vi "picoquant_datalog_loop.vi"(8 "error in (no error)":errorcluster, 11 "picoquant_generic in":refnum<class "picoquant_generic.lvclass">) -> (0 "error out":errorcluster, 3 "picoquant_generic out":refnum<class "picoquant_generic.lvclass">)   [LabVIEW 2015, in "picoquant_generic.lvclass"]
uses:
  picoquant_generic.lvclass
  picoquant_generic.lvclass/picoquant_generic.ctl
  loop_notifier_tdef.ctl
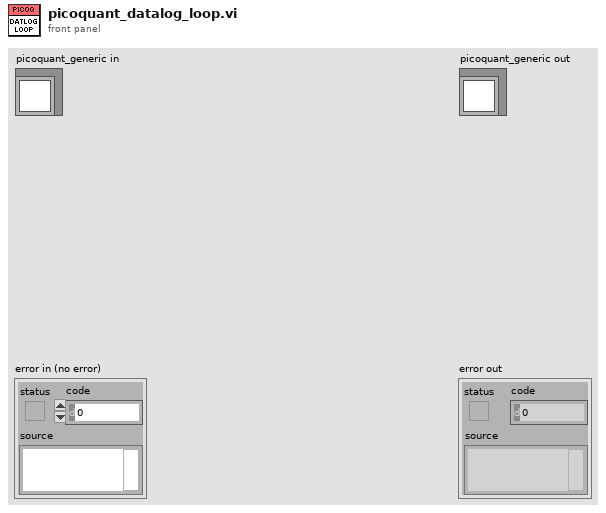
[diagram p1: front panel]
types:
  T1 = typedef "loop_notifier_tdef.ctl" = enum16{"exit"}
  T2 = typedef "picoquant_data_tdef.ctl" = cluster{"channels":u8[], "times":u64[], "sync":u64[]}
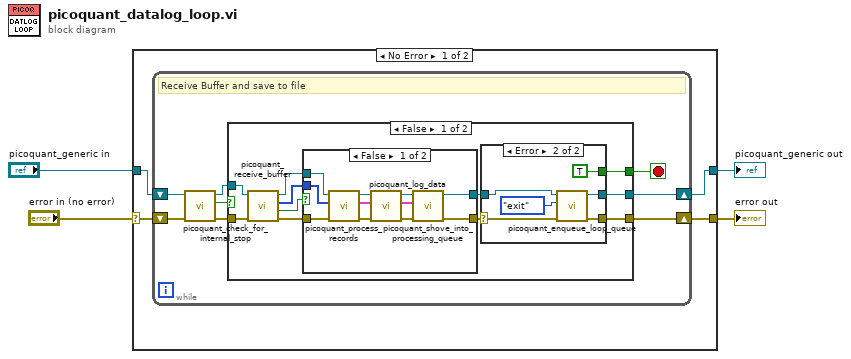
[diagram p0: block diagram]
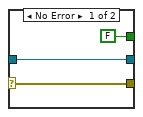
[diagram p2: hidden frame]
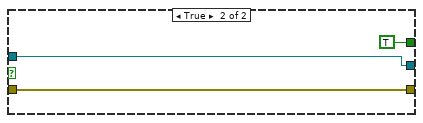
[diagram p4: hidden frame]
diagram:
  n1 = case shown="No Error" "error in (no error)" {
    selector: "error in (no error)" -> [w7 w54]
    tunnel: [w6 w54] -> w3
    tunnel: [w5 w53] -> w1
    tunnel: "picoquant_generic in" -> [w8 w53]
    frame No Error {
      n2 = while {
        shift-right: [w11] -> w5
        shift-left: w8 -> [w15]
        shift-right: [w10] -> w6
        shift-left: w7 -> [w16]
        stop <- w9 stop-if-true
        # "Receive Buffer and save to file"
        n3 = call "picoquant_check_for_internal_stop.vi"("error in (no error)"=w16, "picoquant_generic in"=w15) -> ("error out"=w13:errorcluster, "exit?"=w14:bool, "picoquant_generic out"=w12:refnum<class "picoquant_generic.lvclass">)  [unwired: 7 in]
        n4 = case shown="False" w14 {
          tunnel: w13 -> [w27 w51]
          tunnel: w12 -> [w26 w52]
          tunnel: [w17 w52] -> w11
          tunnel: [w19 w51] -> w10
          tunnel: [w18 TRUE] -> w9
          frame False {
            n5 = call "picoquant_receive_buffer.vi"("error in (no error)"=w27, "picoquant_generic in"=w26) -> ("error out"=w23:errorcluster, "queue_timed_out"=w25:bool, "data"=w22:u32[], "picoquant_generic out"=w24:refnum<class "picoquant_generic.lvclass">)  [unwired: 6 in]
            n6 = case shown="False" w25 {
              tunnel: w24 -> [w47 w49]
              tunnel: [w39 w49] -> w20
              tunnel: w23 -> [w45 w48]
              tunnel: [w38 w48] -> w21
              tunnel: w22 -> [w46 _]
              frame False {
                n7 = call-dynamic "picoquant_process_records.vi"("error in (no error)"=w45, "data"=w46, "picoquant_generic in"=w47) -> ("error out"=w44:errorcluster, "data 2"=w42:T2, "picoquant_generic out"=w43:refnum<class "picoquant_generic.lvclass">)  [unwired: 6 in]
                n8 = call-dynamic "picoquant_log_data.vi"("error in (no error)"=w44, "data_in"=w42, "picoquant_generic in"=w43) -> ("error out"=w41:errorcluster, "data_out"=w37:T2, "picoquant_generic out"=w40:refnum<class "picoquant_generic.lvclass">)  [unwired: 6 in]
                n9 = call "picoquant_shove_into_processing_queue.vi"("error in (no error)"=w41, "data_in"=w37, "picoquant_generic in"=w40) -> ("error out"=w38:errorcluster, "picoquant_generic out"=w39:refnum<class "picoquant_generic.lvclass">)  [unwired: 7 in]
              }
              frame True {
              }
            }
            n10 = case shown="Error" w21 {
              selector: w21 -> [w30 w34]
              tunnel: w20 -> [w28 w36]
              tunnel: [w30 w31] -> w19
              tunnel: [FALSE TRUE] -> w18
              tunnel: [w28 w32] -> w17
              frame No Error {
              }
              frame Error {
                n11 = call "picoquant_enqueue_loop_queue.vi"("error in (no error)"=w34, "loop_notifier"=loop_notifier_tdef."exit" ("element"), "picoquant_generic in"=w36) -> ("error out"=w31:errorcluster, "picoquant_generic out"=w32:refnum<class "picoquant_generic.lvclass">)  [unwired: 7 in]
              }
            }
          }
          frame True {
          }
        }
      }
    }
    frame Error {
    }
  }
  "error out" <- w3
  "picoquant_generic out" <- w1
